vi "Vibration.vi"() -> ()   [LabVIEW 2012]
uses:
  <vilib>/Analysis/NI_AALPro.lvlib
panel:
  out "选项卡":T1(tab)
  in  "装置IP":string
  in  "?":bool
  in  "采样率(ksps)":T2(ring)=enum."105.468"
  in  "?":bool
  in  "?":bool
  in  "开始":bool
  in  "?":bool
  in  "设置装置网关":string
  in  "设置装置子网掩码":string
  in  "设置装置IP":string
  in  "?":bool
  in  "是否开启电流源":u8(knob)=1 scale=0.0..1.0
  in  "是否进行自校准":u8(knob) scale=0.0..1.0
  in  "?":bool
  in  "?":path
  in  "是否保存数据":u8(knob) scale=0.0..1.0
  in  "?":bool
  out "进度条":dbl(slide) scale=0.0..99.0
  out "字符串":string
  out "波形卡":enum32{"波形卡 1", "波形卡 2", "波形卡 3"}(tab)
  in  "AC/DC":bool
  in  "Y轴调整":dbl(knob)=5000.0 min=1.0 max=5000.0 step=1.0 scale=1.0..5000.0 scale format="%#_1g"
  out "?":dbl[][](graph)
  out "?":dbl[][](graph)
  in  "X轴调整":u32(knob)=50000 min=1000 max=50000 step=100 scale=1100.0..50000.0
  in  "通道1":bool=TRUE
  in  "通道2":bool=TRUE
  in  "通道3":bool=TRUE
  in  "通道4":bool=TRUE
  in  "灵敏度1(mv/g)":i32=1 min=1
  in  "灵敏度2(mv/g)":i32=1 min=1
  in  "灵敏度3(mv/g)":i32=1 min=1
  in  "灵敏度4(mv/g)":i32=1 min=1
  out "?":u16[](graph)
  out "转 \n速":u16(knob) scale=0.0..20000.0
  # "PageUp\nPageDown\n微调"
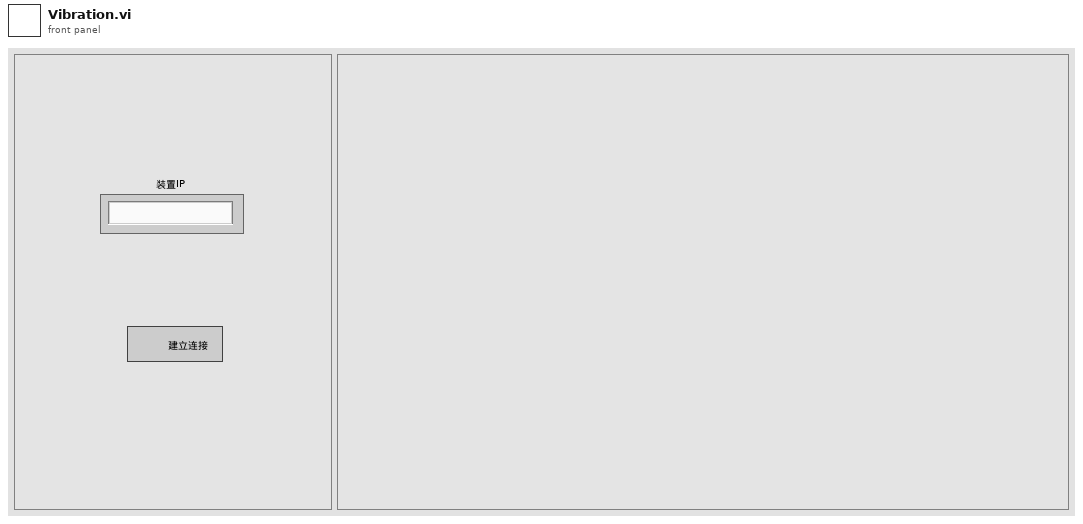
[diagram p1: front panel]
types:
  T1 = enum32{"选项卡 1", "选项卡 2", "选项卡 3", "选项卡 4", "选项卡 5", "选项卡 6", "选项卡 7"}
  T2 = enum16{"", "105.468", "52.734", "35.156", "26.367", "21.094", "17.578", "15.067", "13.184", "11.719", "10.545"}
  T3 = enum8{"Enabled", "Disabled", "Disabled and Grayed Out"}
  T4 = cluster{"refnum":refnum<file>, "refnum":refnum<file>, "refnum":refnum<file>, "refnum":refnum<file>, "refnum":refnum<file>, "SavePath":path, "SAVE?":bool, "connection ID":refnum<k5>}
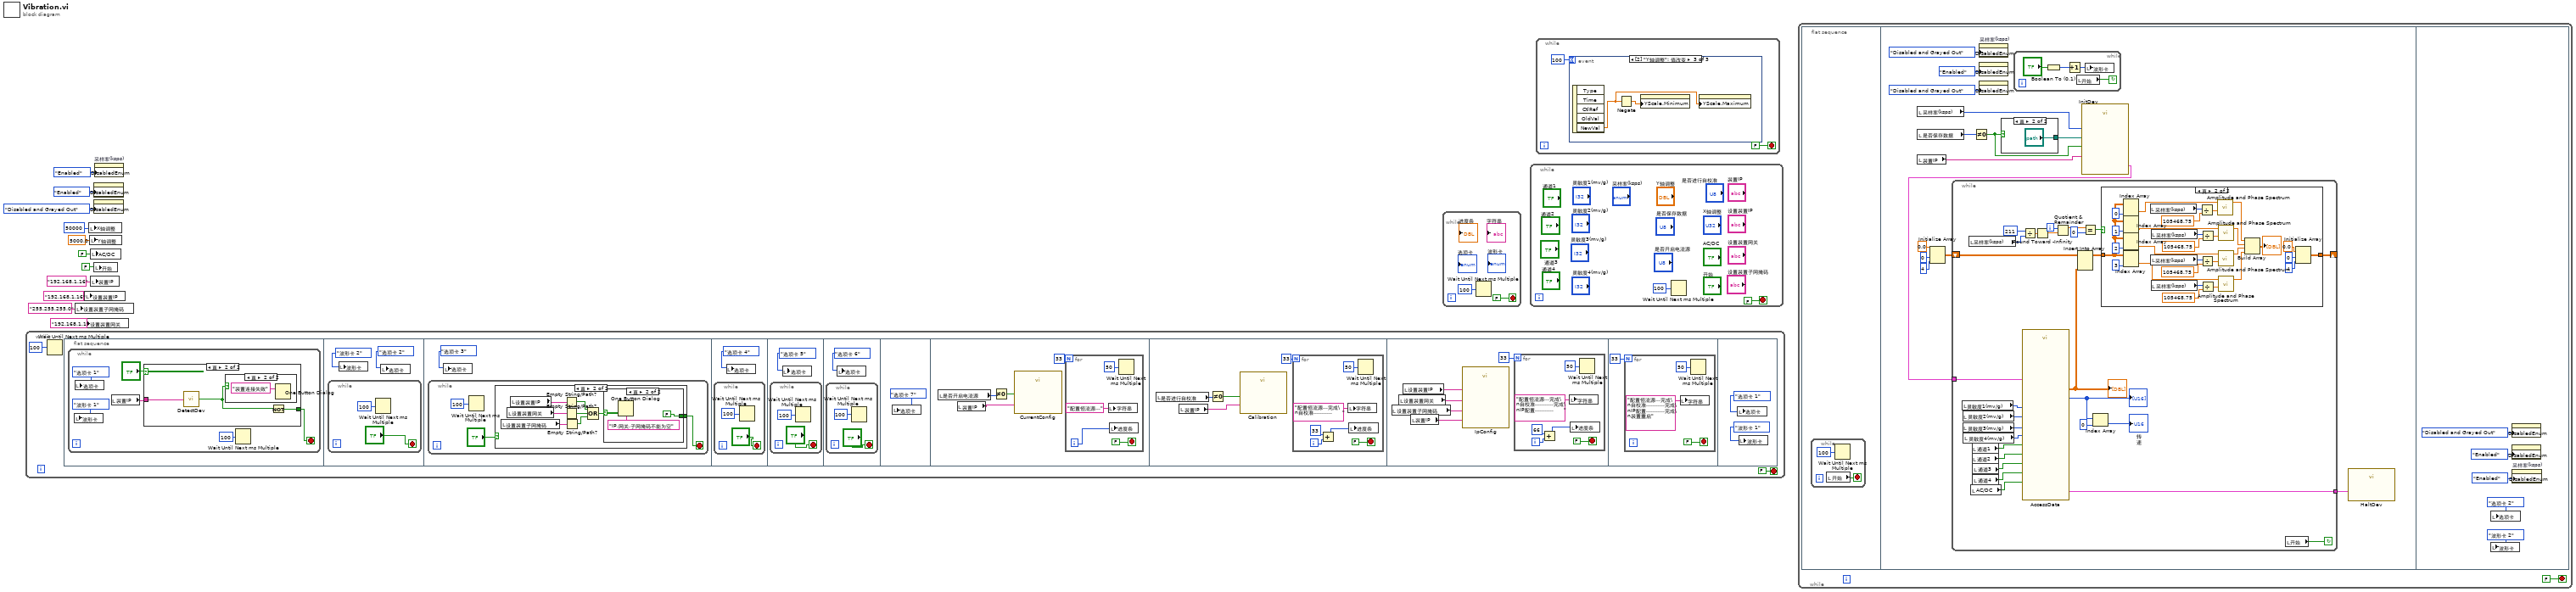
[diagram p0: block diagram]
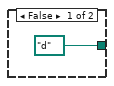
[diagram p3: hidden frame]
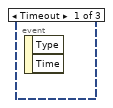
[diagram p4: hidden frame]
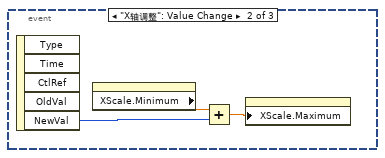
[diagram p5: hidden frame]
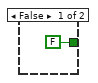
[diagram p6: hidden frame]
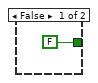
[diagram p8: hidden frame]
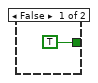
[diagram p9: hidden frame]
diagram:
  n1 = while {
    stop <- FALSE stop-if-true
    n2 = Wait Until Next ms Multiple(millisecond multiple=u32 100 ("毫秒倍数")) -> ()  [unwired: 1 out]
    n3 = flat-sequence {
      frame #0 {
        n4 = while {
          stop <- w18 stop-if-true
          n5 = local write "波形卡"(enum32{"波形卡 1", "波形卡 2", "波形卡 3"}."波形卡 1" ("波形卡")) -> ()
          n6 = local write "选项卡"(T1."选项卡 1" ("选项卡")) -> ()
          n7 = local read "装置IP"() -> (w14:string)
          n8 = case shown="真" "?" {
            tunnel: [FALSE w23] -> w18
            tunnel: w14 -> [_ w21]
            frame False {
            }
            frame True {
              n9 = call "DetectDev.vi"("IP."=w21) -> ("Fail"=w22:bool)
              n10 = case shown="真" w22 {
                frame False {
                }
                frame True {
                  n11 = One Button Dialog(message="装置连接失败" ("消息")) -> ()  [unwired: 1 in, 1 out]
                }
              }
              n12 = Not(x=w22) -> (.not. x?=w23:bool)
            }
          }
          n13 = Wait Until Next ms Multiple(millisecond multiple=u32 100 ("毫秒倍数")) -> ()  [unwired: 1 out]
        }
      }
      frame #1 {
        n14 = while {
          stop <- "?" stop-if-true
          n15 = Wait Until Next ms Multiple(millisecond multiple=u32 100 ("毫秒倍数")) -> ()  [unwired: 1 out]
        }
        n16 = local write "波形卡"(enum32{"波形卡 1", "波形卡 2", "波形卡 3"}."波形卡 2" ("波形卡")) -> ()
        n17 = local write "选项卡"(T1."选项卡 2" ("选项卡")) -> ()
      }
      frame #2 {
        n18 = while {
          stop <- w30 stop-if-true
          n19 = Wait Until Next ms Multiple(millisecond multiple=u32 100 ("毫秒倍数")) -> ()  [unwired: 1 out]
          n20 = case shown="真" "?" {
            tunnel: [FALSE w34] -> w30
            frame False {
            }
            frame True {
              n21 = local read "设置装置子网掩码"() -> (w41:string)
              n22 = local read "设置装置网关"() -> (w40:string)
              n23 = local read "设置装置IP"() -> (w39:string)
              n24 = Empty String/Path?(string/path=w39) -> (empty?=w36:bool)
              n25 = Empty String/Path?(string/path=w40) -> (empty?=w37:bool)
              n26 = Empty String/Path?(string/path=w41) -> (empty?=w38:bool)
              n27 = Compound Arithmetic op=OR(w36, w37, w38) -> (w35:bool)
              n28 = case shown="真" w35 {
                tunnel: [TRUE FALSE] -> w34
                frame False {
                }
                frame True {
                  n29 = One Button Dialog(message="IP,网关,子网掩码不能为空" ("消息")) -> ()  [unwired: 1 in, 1 out]
                }
              }
            }
          }
        }
        n30 = local write "选项卡"(T1."选项卡 3" ("选项卡")) -> ()
      }
      frame #3 {
        n31 = while {
          stop <- "?" stop-if-true
          n32 = Wait Until Next ms Multiple(millisecond multiple=u32 100 ("毫秒倍数")) -> ()  [unwired: 1 out]
        }
        n33 = local write "选项卡"(T1."选项卡 4" ("选项卡")) -> ()
      }
      frame #4 {
        n34 = while {
          stop <- "?" stop-if-true
          n35 = Wait Until Next ms Multiple(millisecond multiple=u32 100 ("毫秒倍数")) -> ()  [unwired: 1 out]
        }
        n36 = local write "选项卡"(T1."选项卡 5" ("选项卡")) -> ()
      }
      frame #5 {
        n37 = while {
          stop <- "?" stop-if-true
          n38 = Wait Until Next ms Multiple(millisecond multiple=u32 100 ("毫秒倍数")) -> ()  [unwired: 1 out]
        }
        n39 = local write "选项卡"(T1."选项卡 6" ("选项卡")) -> ()
      }
      frame #6 {
        n40 = local write "选项卡"(T1."选项卡 7" ("选项卡")) -> ()
      }
      frame #7 {
        n41 = local read "是否开启电流源"() -> (w56:u8)
        n42 = local read "装置IP"() -> (w55:string)
        n43 = Not Equal To 0?(x=w56) -> (x != 0?=w57:bool)
        n44 = call "CurrentConfig.vi"("Current"=w57, "IP"=w55) -> ()
        n45 = for {
          N: 33 -> [_]
          i -> [w59]
          stop <- FALSE stop-if-true
          n46 = local write "字符串"("配置恒流源..." ("字符串")) -> ()
          n47 = local write "进度条"(w59) -> ()
          n48 = Wait Until Next ms Multiple(millisecond multiple=u32 50 ("毫秒倍数")) -> ()  [unwired: 1 out]
        }
      }
      frame #8 {
        n49 = local read "是否进行自校准"() -> (w64:u8)
        n50 = local read "装置IP"() -> (w63:string)
        n51 = Not Equal To 0?(x=w64) -> (x != 0?=w65:bool)
        n52 = call "Calibration.vi"("Enable"=w65, "IP."=w63) -> ()
        n53 = for {
          N: 33 -> [_]
          i -> [w69]
          stop <- FALSE stop-if-true
          n54 = Add(x=33, y=w69) -> (x+y=w68:i32)
          n55 = local write "字符串"("配置恒流源...完成\n自校准...........      " ("字符串")) -> ()
          n56 = local write "进度条"(w68) -> ()
          n57 = Wait Until Next ms Multiple(millisecond multiple=u32 50 ("毫秒倍数")) -> ()  [unwired: 1 out]
        }
      }
      frame #9 {
        n58 = local read "设置装置子网掩码"() -> (w75:string)
        n59 = local read "设置装置网关"() -> (w74:string)
        n60 = local read "设置装置IP"() -> (w73:string)
        n61 = local read "装置IP"() -> (w76:string)
        n62 = call "IpConfig.vi"("Gateway"=w74, "SubnetMask"=w75, "IP"=w73, "CurrentIP"=w76) -> ()
        n63 = for {
          N: 33 -> [_]
          i -> [w80]
          stop <- FALSE stop-if-true
          n64 = Add(x=66, y=w80) -> (x+y=w79:i32)
          n65 = local write "字符串"("配置恒流源...完成\n自校准...........完成\nIP配置...........      " ("字符串")) -> ()
          n66 = local write "进度条"(w79) -> ()
          n67 = Wait Until Next ms Multiple(millisecond multiple=u32 50 ("毫秒倍数")) -> ()  [unwired: 1 out]
        }
      }
      frame #10 {
        n68 = for {
          N: 33 -> [_]
          stop <- FALSE stop-if-true
          n69 = local write "字符串"("配置恒流源...完成\n自校准...........完成\nIP配置...........完成\n装置重启" ("字符串")) -> ()
          n70 = Wait Until Next ms Multiple(millisecond multiple=u32 50 ("毫秒倍数")) -> ()  [unwired: 1 out]
        }
      }
      frame #11 {
        n71 = local write "选项卡"(T1."选项卡 1" ("选项卡")) -> ()
        n72 = local write "波形卡"(enum32{"波形卡 1", "波形卡 2", "波形卡 3"}."波形卡 1" ("波形卡")) -> ()
      }
    }
  }
  n73 = local write "设置装置子网掩码"("255.255.255.0" ("新子网掩码")) -> ()
  n74 = local write "设置装置网关"("192.168.1.1" ("新网关")) -> ()
  n75 = local write "设置装置IP"("192.168.1.16" ("新装置IP")) -> ()
  n76 = local write "X轴调整"(u16 50000 ("X轴调整")) -> ()
  n77 = local write "Y轴调整"(5000.0 ("Y轴调整")) -> ()
  n78 = local write "AC/DC"(FALSE ("AC/DC")) -> ()
  n79 = local write "装置IP"("192.168.1.16" ("装置IP")) -> ()
  n80 = property class="Bool"("DisabledEnum"=T3."Enabled" ("禁用")) -> ()  [unwired: 2 in, 2 out]
  n81 = property class="Bool (严格)"("DisabledEnum"=T3."Disabled and Grayed Out" ("禁用")) -> ()  [unwired: 2 in, 2 out]
  n82 = local write "开始"(FALSE ("开始")) -> ()
  n83 = property on="采样率(ksps)" class="Enum (严格)"("DisabledEnum"=T3."Enabled" ("禁用")) -> ()  [unwired: 2 in, 2 out]
  n84 = while {
    stop <- FALSE stop-if-true
    n85 = Wait Until Next ms Multiple(millisecond multiple=u32 100 ("毫秒倍数")) -> ()  [unwired: 1 out]
  }
  n86 = while {
    stop <- FALSE stop-if-true
    n87 = Wait Until Next ms Multiple(millisecond multiple=u32 100 ("毫秒倍数")) -> ()  [unwired: 1 out]
  }
  n88 = while {
    stop <- FALSE stop-if-true
    n89 = event shown="[2] \"Y轴调整\": 值改变" {
      selector: _ -> [_ _ _]
      dyn-events: _ -> [_ _ _]
      timeout: 100 -> [_ _ _]
      event Timeout {
        n90 = event-data() -> ()  [unwired: 1 in, 2 out]
      }
      event "X轴调整": Value Change {
        n91 = event-data() -> ("NewVal"=w98:u32)  [unwired: 1 in, 4 out]
        n92 = property class="WFChart (严格)"() -> ("XScale.Minimum"=w97:dbl)  [unwired: 2 in, 2 out]
        n93 = Add(x=w97, y=w98) -> (x+y=w96:dbl)
        n94 = property class="WFChart (严格)"("XScale.Maximum"=w96) -> ()  [unwired: 2 in, 2 out]
      }
      event "Y轴调整": Value Change {
        n95 = event-data() -> ("NewVal"=w99:dbl)  [unwired: 1 in, 4 out]
        n96 = Negate(x=w99) -> (-x=w100:dbl)
        n97 = property class="WFChart (严格)"("YScale.Minimum"=w100) -> ()  [unwired: 2 in, 2 out]
        n98 = property class="WFChart (严格)"("YScale.Maximum"=w99) -> ()  [unwired: 2 in, 2 out]
      }
    }
  }
  n99 = while {
    stop <- FALSE stop-if-true
    n100 = flat-sequence {
      frame #0 {
        n101 = while {
          stop <- w102 stop-if-true
          n102 = local read "开始"() -> (w102:bool)
          n103 = Wait Until Next ms Multiple(millisecond multiple=u32 100 ("毫秒倍数")) -> ()  [unwired: 1 out]
        }
      }
      frame #1 {
        n104 = local read "采样率(ksps)"() -> (w105:T2)
        n105 = local read "是否保存数据"() -> (w117:u8)
        n106 = local read "装置IP"() -> (w112:string)
        n107 = Initialize Array(0.0 ("元素"), 0 ("维数大小"), 4 ("维数大小")) -> (w106:dbl[][])
        n108 = Not Equal To 0?(x=w117) -> (x != 0?=w113:bool)
        n109 = property on="采样率(ksps)" class="Enum (严格)"("DisabledEnum"=T3."Disabled and Grayed Out" ("禁用")) -> ()  [unwired: 2 in, 2 out]
        n110 = property class="Bool (严格)"("DisabledEnum"=T3."Enabled" ("禁用")) -> ()  [unwired: 2 in, 2 out]
        n111 = property class="Bool"("DisabledEnum"=T3."Disabled and Grayed Out" ("禁用")) -> ()  [unwired: 2 in, 2 out]
        n112 = case shown="真" w113 {
          tunnel: [path "d:/" ("路径（使用对话框）") "?"] -> w114
          frame False {
          }
          frame True {
          }
        }
        n113 = while {
          stop <- w176 continue-if-true
          n114 = Boolean To (0,1)(Boolean="?") -> (0, 1=w179:i16)
          n115 = Increment(x=w179) -> (x+1=w177:i16)
          n116 = local read "开始"() -> (w176:bool)
          n117 = local write "波形卡"(w177) -> ()
        }
        n118 = call "InitDev.vi"("SAVE?"=w113, "IP地址"=w112, "SampleRate"=w105, "SavePath"=w114) -> ("输出簇"=w111:T4)
        n119 = while {
          tunnel: w111 -> [w141]
          tunnel: [w140] -> w110
          shift-right: [w136] -> _
          shift-left: w106 -> [w138]
          i -> [w133]
          stop <- w142 continue-if-true
          n120 = local read "灵敏度1(mv/g)"() -> (w126:i32)
          n121 = local read "灵敏度2(mv/g)"() -> (w125:i32)
          n122 = local read "灵敏度3(mv/g)"() -> (w124:i32)
          n123 = local read "灵敏度4(mv/g)"() -> (w123:i32)
          n124 = local read "采样率(ksps)"() -> (w130:T2)
          n125 = local read "AC/DC"() -> (w118:bool)
          n126 = local read "通道1"() -> (w122:bool)
          n127 = local read "通道2"() -> (w121:bool)
          n128 = local read "通道3"() -> (w120:bool)
          n129 = local read "通道4"() -> (w119:bool)
          n130 = call "AccessData.vi"("Sensitivity1"=w126, "CH1Enable"=w122, "Sensitivity2"=w125, "CH2Enable"=w121, "Sensitivity3"=w124, "CH3Enable"=w120, "Sensitivity4"=w123, "CH4Enable"=w119, "输入簇"=w141, "RmOffset"=w118) -> ("VibrationWave"=w127:dbl[][], "Speed"=w139:u16[], "输出簇"=w140:T4)  [unwired: 2 in, 1 out]
          "?" <- w127
          "?" <- w139
          n131 = Divide(x=u8 211, y=w130) -> (x/y=w131:dbl)
          n132 = Round Toward -Infinity(1:w131) -> (0:w129:dbl)
          n133 = Quotient & Remainder(x=w133, y=w129) -> (x-y*floor(x/y)=w135:dbl)  [unwired: 1 out]
          n134 = Insert Into Array(array=w138, new element=w127) -> (w137:dbl[][])  [unwired: 2 in]
          n135 = Equal?(x=w135, y=0) -> (x = y?=w128:bool)
          n136 = Index Array(array=w139, index=0 ("索引")) -> (element=→"转 \n速":u16)
          n137 = case shown="真" w128 {
            tunnel: w137 -> [w145 w152]
            tunnel: [w145 w148] -> w136
            frame False {
            }
            frame True {
              n138 = Index Array(array=w152, index (col)=0 ("禁用的索引 (列)")) -> (element=w154:dbl[])  [unwired: 1 in]
              n139 = Index Array(array=w152, index (col)=1 ("禁用的索引 (列)")) -> (element=w161:dbl[])  [unwired: 1 in]
              n140 = Index Array(array=w152, index (col)=2 ("禁用的索引 (列)")) -> (element=w160:dbl[])  [unwired: 1 in]
              n141 = Index Array(array=w152, index (col)=3 ("禁用的索引 (列)")) -> (element=w159:dbl[])  [unwired: 1 in]
              n142 = local read "采样率(ksps)"() -> (w171:T2)
              n143 = local read "采样率(ksps)"() -> (w165:T2)
              n144 = local read "采样率(ksps)"() -> (w168:T2)
              n145 = local read "采样率(ksps)"() -> (w162:T2)
              n146 = Divide(x=w171, y=105468.75 ("dt")) -> (x/y=w146:dbl)
              n147 = Divide(x=w165, y=105468.75 ("dt")) -> (x/y=w166:dbl)
              n148 = Divide(x=w168, y=105468.75 ("dt")) -> (x/y=w169:dbl)
              n149 = Divide(x=w162, y=105468.75 ("dt")) -> (x/y=w163:dbl)
              n150 = call <vilib>:"Amplitude and Phase Spectrum.vi"("dt"=w146, "Signal (V)"=w154) -> ("Amp Spectrum Mag (Vrms)"=w158:dbl[])  [unwired: 1 in, 2 out]
              n151 = call <vilib>:"Amplitude and Phase Spectrum.vi"("dt"=w166, "Signal (V)"=w160) -> ("Amp Spectrum Mag (Vrms)"=w155:dbl[])  [unwired: 1 in, 2 out]
              n152 = call <vilib>:"Amplitude and Phase Spectrum.vi"("dt"=w169, "Signal (V)"=w161) -> ("Amp Spectrum Mag (Vrms)"=w157:dbl[])  [unwired: 1 in, 2 out]
              n153 = call <vilib>:"Amplitude and Phase Spectrum.vi"("dt"=w163, "Signal (V)"=w159) -> ("Amp Spectrum Mag (Vrms)"=w156:dbl[])  [unwired: 1 in, 2 out]
              n154 = Build Array(w158, w157, w155, w156) -> (→"?":dbl[][])
              n155 = Initialize Array(0.0 ("元素"), 0 ("维数大小"), 4 ("维数大小")) -> (w148:dbl[][])
            }
          }
          n156 = local read "开始"() -> (w142:bool)
        }
        n157 = call "HaltDev.vi"("输入簇"=w110) -> ()
      }
      frame #2 {
        n158 = local write "波形卡"(enum32{"波形卡 1", "波形卡 2", "波形卡 3"}."波形卡 2" ("波形卡")) -> ()
        n159 = local write "选项卡"(T1."选项卡 2" ("选项卡")) -> ()
        n160 = property class="Bool (严格)"("DisabledEnum"=T3."Disabled and Grayed Out" ("禁用")) -> ()  [unwired: 2 in, 2 out]
        n161 = property class="Bool"("DisabledEnum"=T3."Enabled" ("禁用")) -> ()  [unwired: 2 in, 2 out]
        n162 = property on="采样率(ksps)" class="Enum (严格)"("DisabledEnum"=T3."Enabled" ("禁用")) -> ()  [unwired: 2 in, 2 out]
      }
    }
  }
